vi "OpenSwerveDrive.vi"(6 "error in":errorcluster, 7 "Ramp Rate":dbl=50.0, 8 "Speed PID":cluster{"P":dbl, "I":dbl, "D":dbl}={"P"=48.0, "I"=0.0, "D"=638.0}, 9 "Steering PID":cluster{"P":dbl, "I":dbl, "D":dbl}={"P"=0.0275, "I"=0.000115, "D"=0.682955}) -> (0 "error out":errorcluster, 2 "Speed Motor Refs":T1[](array[typedef]), 3 "Steering Motor Refs":T1[](array[typedef]))   [LabVIEW 2015, in "Team900SwerveDrive.lvlib"]
uses:
  Team900SwerveDrive.lvlib
  <vilib>/Rock Robotics/WPI/MotorControl/WPI_MotorControlDeviceRef.ctl
  <vilib>/Rock Robotics/WPI/MotorControl/WPI_MotorControlType.ctl
  <vilib>/Rock Robotics/SystemInterfaces/DIO/FPGA_DIOPWMChannel.ctl
  <vilib>/Rock Robotics/WPI/PWM/WPI_PWMDeadband.ctl
  <vilib>/Rock Robotics/WPI/CAN/Jaguar/SubVIs/WPI_CANJaguar_ControlMode.ctl
  <vilib>/Rock Robotics/WPI/CAN/TalonSRX/WPI_CANTalonSRX_APIControlMode.ctl
  <vilib>/Rock Robotics/WPI/MotorControl/WPI_MotorControlOpenCANTalonSRX.vi
  SwerveGlobalData.vi
  <vilib>/Rock Robotics/WPI/CAN/TalonSRX/WPI_CANTalonSRX_APIFeedbackSelect.ctl
panel:
  # "This should be run in Begin.vi. No inputs are needed,\nalthough there are terminals for PID values.\nThe motor controllers should have the following ID\nvalues:\nFL Steering: 11\nFR Steering: 12\nRL Steering: 13\nRR Steering: 14\nFL Speed: 21\nFR Speed: 22\nRL Speed: 23\nRR Speed: 24"
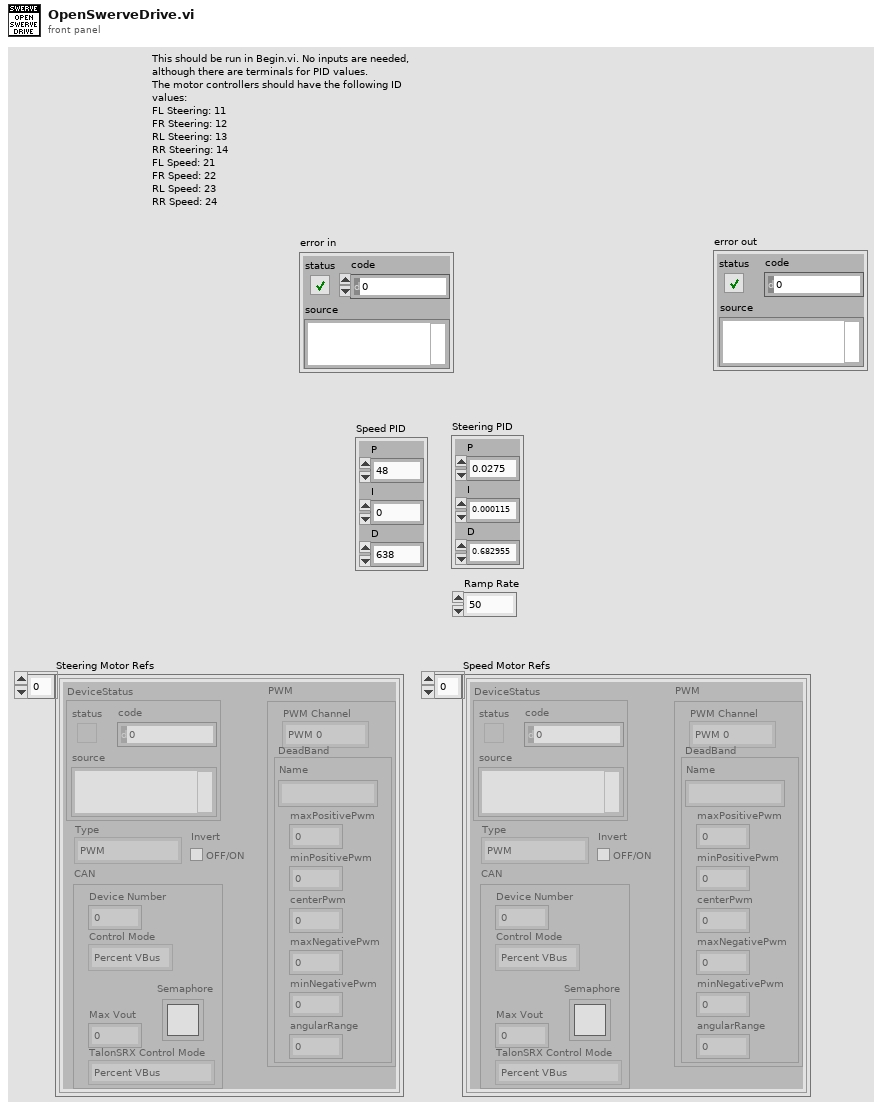
[diagram p1: front panel]
types:
  T1 = typedef "WPI_MotorControlDeviceRef.ctl" = cluster{"DeviceStatus":errorcluster, "Type":T2, "PWM":cluster{"PWM Channel":T3, "DeadBand":T4}, "CAN":cluster{"Device Number":u8, "Control Mode":T5, "Semaphore":T6, "Max Vout":dbl, "TalonSRX Control Mode":T7}, "Invert":bool}
  T2 = typedef "WPI_MotorControlType.ctl" = enum16{"PWM", "CAN", "CANTalonSRX"}
  T3 = typedef "FPGA_DIOPWMChannel.ctl" = enum8{"PWM 0", "PWM 1", "PWM 2", "PWM 3", "PWM 4", "PWM 5", "PWM 6", "PWM 7", "PWM 8", "PWM 9", "PWM MXP 0", "PWM MXP 1", "PWM MXP 2", "PWM MXP 3", "PWM MXP 4", "PWM MXP 5", "PWM MXP 6", "PWM MXP 7", "PWM MXP 8", "PWM MXP 9", "Invalid"}
  T4 = typedef "WPI_PWMDeadband.ctl" = cluster{"Name":string, "maxPositivePwm":i32, "minPositivePwm":i32, "centerPwm":i32, "maxNegativePwm":i32, "minNegativePwm":i32, "angularRange":u16}
  T5 = typedef "WPI_CANJaguar_ControlMode.ctl" = enum8{"Percent VBus", "Current", "Speed", "Position", "Voltage"}
  T6 = typedef "Semaphore RefNum" = refnum<k1>
  T7 = typedef "WPI_CANTalonSRX_APIControlMode.ctl" = enum8{"Percent VBus", "Speed", "Position", "Slave", "Unchanged / Invalid", "Voltage Compensation", "Current", "Motion Profile"}
  T8 = typedef "WPI_CANTalonSRX_APIFeedbackSelect.ctl" = enum16{"Digital Quadrature Encoder", "Analog Potentiometer", "Analog Encoder", "Count on Quad-A (Rising-Edge)", "Count on Quad-A (Falling-Edge)", "CTR Magnetic Enc (Absolute)", "CTR Magnetic Enc (Relative)", "Pulse Width"}
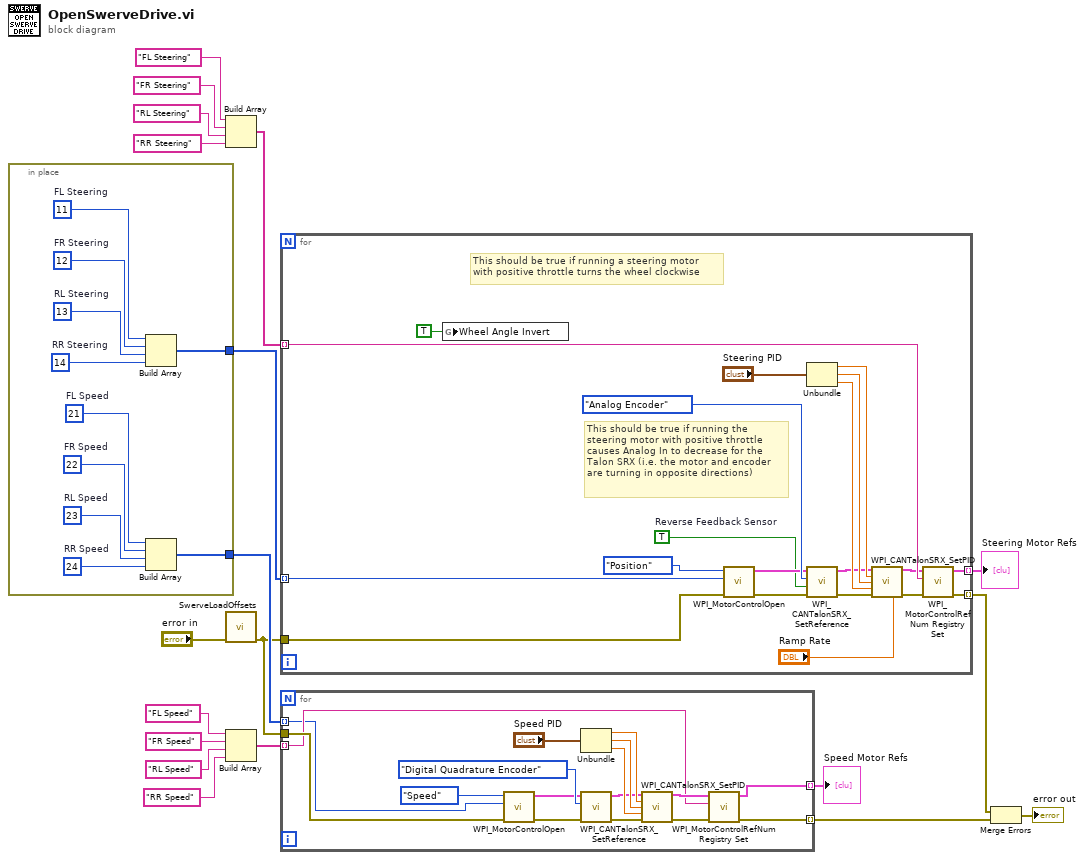
[diagram p0: block diagram]
diagram:
  n1 = in-place {
    in-place-border: [w25] -> w17
    in-place-border: [w20] -> w5
    w29 = u8 11  # FL Steering
    w21 = u8 24  # RR Speed
    w22 = u8 23  # RL Speed
    w23 = u8 22  # FR Speed
    w24 = u8 21  # FL Speed
    w26 = u8 14  # RR Steering
    w27 = u8 13  # RL Steering
    w28 = u8 12  # FR Steering
    n2 = Build Array(w29, w28, w27, w26) -> (w25:u8[])
    n3 = Build Array(w24, w23, w22, w21) -> (w20:u8[])
  }
  n4 = Build Array("FL Steering" ("refnum name"), "FR Steering" ("refnum name"), "RL Steering" ("refnum name"), "RR Steering" ("refnum name")) -> (w12:string[])
  n5 = call "SwerveLoadOffsets.vi"("error in (no error)"="error in") -> ("error out"=w3:errorcluster)  [unwired: 10 in]
  n6 = Build Array("FL Speed" ("refnum name"), "FR Speed" ("refnum name"), "RL Speed" ("refnum name"), "RR Speed" ("refnum name")) -> (w6:string[])
  n7 = for {
    tunnel: w3 -> [w46]
    tunnel: [w41] -> w11 mode=indexing
    tunnel: w17 -> [w40] mode=indexing
    tunnel: w12 -> [w39] mode=indexing
    tunnel: [w30] -> w1 mode=indexing
    w32 = TRUE  # Reverse Feedback Sensor
    # "This should be true if running the\nsteering motor with positive throttle\ncauses Analog In to decrease for the\nTalon SRX (i.e. the motor and encoder\nare turning in opposite directions)"
    # "This should be true if running a steering motor \nwith positive throttle turns the wheel clockwise"
    n8 = global write "SwerveGlobalData.vi" "Wheel Angle Invert"(TRUE ("Drive Train Invert")) -> ()
    n9 = call-poly <vilib>:"WPI_MotorControlOpen.vi"("error in (no error)"=w46, "Device Number"=w40, "Control Mode"=WPI_CANTalonSRX_APIControlMode."Position") -> ("error out"=w42:errorcluster, "MotorControlDeviceRef"=w36:T1)  [unwired: 7 in]
    n10 = Unbundle("Steering PID") -> ("P"=w49:dbl, "I"=w48:dbl, "D"=w47:dbl)
    n11 = call <vilib>:"WPI_CANTalonSRX_SetReference.vi"("error in (no error)"=w42, "Reverse Feedback Sensor"=w32, "Feedback Reference"=WPI_CANTalonSRX_APIFeedbackSelect."Analog Encoder", "CAN Talon SRX Ref"=w36) -> ("error out"=w45:errorcluster, "CAN Talon SRX Ref"=w44:T1)  [unwired: 6 in]
    n12 = call <vilib>:"WPI_CANTalonSRX_SetPID.vi"("CAN Talon SRX Ref"=w44, "P"=w49, "I"=w48, "D"=w47, "error in (no error)"=w45, "Ramp Rate"="Ramp Rate") -> ("CAN Talon SRX Ref"=w34:T1, "error out"=w33:errorcluster)  [unwired: 8 in]
    n13 = call <vilib>:"WPI_MotorControlRefNum Registry Set.vi"("error in (no error)"=w33, "refnum name"=w39, "MotorControlDevRef"=w34) -> ("error out"=w41:errorcluster, "MotorControlDevRef"=w30:T1)  [unwired: 7 in]
  }
  "Steering Motor Refs" <- w1
  n14 = for {
    tunnel: w3 -> [w62]
    tunnel: [w59] -> w19 mode=indexing
    tunnel: w6 -> [w54] mode=indexing
    tunnel: w5 -> [w53] mode=indexing
    tunnel: [w50] -> w2 mode=indexing
    n15 = call-poly <vilib>:"WPI_MotorControlOpen.vi"("error in (no error)"=w62, "Device Number"=w53, "Control Mode"=WPI_CANTalonSRX_APIControlMode."Speed") -> ("error out"=w52:errorcluster, "MotorControlDeviceRef"=w51:T1)  [unwired: 7 in]
    n16 = Unbundle("Speed PID") -> ("P"=w65:dbl, "I"=w64:dbl, "D"=w63:dbl)
    n17 = call <vilib>:"WPI_CANTalonSRX_SetReference.vi"("error in (no error)"=w52, "Feedback Reference"=WPI_CANTalonSRX_APIFeedbackSelect."Digital Quadrature Encoder", "CAN Talon SRX Ref"=w51) -> ("error out"=w57:errorcluster, "CAN Talon SRX Ref"=w58:T1)  [unwired: 7 in]
    n18 = call <vilib>:"WPI_CANTalonSRX_SetPID.vi"("CAN Talon SRX Ref"=w58, "P"=w65, "I"=w64, "D"=w63, "error in (no error)"=w57) -> ("CAN Talon SRX Ref"=w60:T1, "error out"=w61:errorcluster)  [unwired: 9 in]
    n19 = call <vilib>:"WPI_MotorControlRefNum Registry Set.vi"("error in (no error)"=w61, "refnum name"=w54, "MotorControlDevRef"=w60) -> ("error out"=w59:errorcluster, "MotorControlDevRef"=w50:T1)  [unwired: 7 in]
  }
  "Speed Motor Refs" <- w2
  n20 = Merge Errors(w11, w19) -> (→"error out":errorcluster)
